vi "GetProperty.vi"(8 "error in (no error)":errorcluster, 10 "key":string, 11 "VeriStandTestCase in":refnum<class "VeriStandTestCase.lvclass">) -> (0 "error out":errorcluster, 2 "value":string, 3 "VeriStandTestCase out":refnum<class "VeriStandTestCase.lvclass">)   [LabVIEW 2027, in "VeriStandTestCase.lvclass"]
uses:
  VeriStandTestCase.lvclass
  VeriStandTestCase.lvclass/VeriStandTestCase.ctl
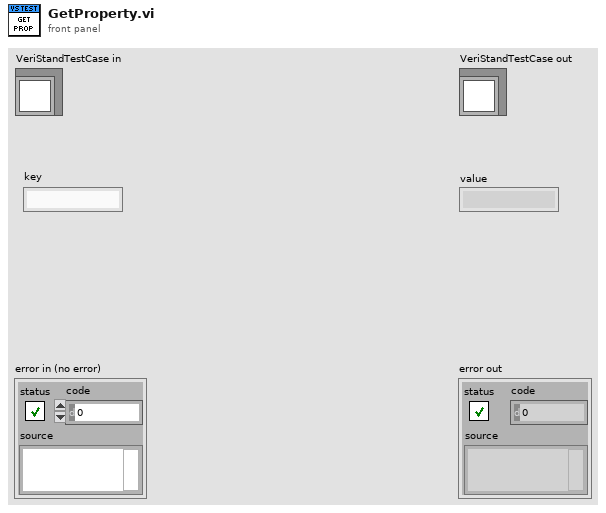
[diagram p1: front panel]
types:
  T1 = typedef "VeriStandTestUtilities.lvlib/ConfigPropertyItem.ctl" = cluster{"key":string, "value":string}
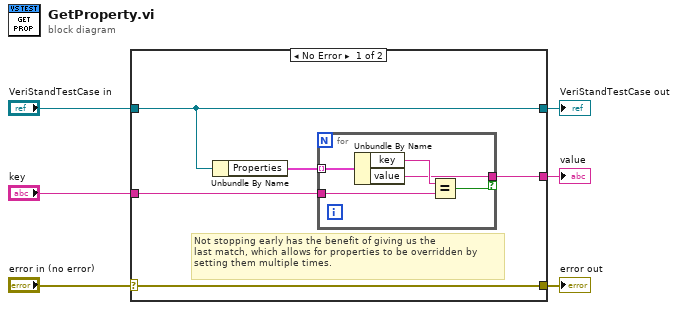
[diagram p0: block diagram]
diagram:
  n1 = case shown="No Error" "error in (no error)" {
    selector: "error in (no error)" -> [w11 w18]
    tunnel: [w11 w18] -> w5
    tunnel: [w10 w17] -> w3
    tunnel: "VeriStandTestCase in" -> [w10 w17]
    tunnel: "key" -> [w8 _]
    tunnel: [w7 _] -> w1
    frame No Error {
      # "Not stopping early has the benefit of giving us the\nlast match, which allows for properties to be overridden by\nsetting them multiple times."
      n2 = Unbundle By Name(w10) -> ("Properties"=w9:T1[])
      n3 = for {
        tunnel: w9 -> [w16] mode=indexing
        tunnel: w8 -> [w14]
        tunnel: [w13] -> w7 if=w12
        n4 = Unbundle By Name(w16) -> ("key"=w15:string, "value"=w13:string)
        n5 = Equal?(x=w15, y=w14) -> (x = y?=w12:bool)
      }
    }
    frame Error {
    }
  }
  "error out" <- w5
  "VeriStandTestCase out" <- w3
  "value" <- w1
